vi "Polarity switch.vi"() -> ()   [LabVIEW 2017]
uses:
  <vilib>/DAQmx/write.llb/DAQmx Write (Digital 1D Bool NChan 1Samp 1Line).vi
  <vilib>/DAQmx/miscellaneous.llb/DAQmx Fill In Error Info.vi
  <instrlib>/Keithley KE22xx Series/Keithley KE22xx Series.lvlib
  <instrlib>/Harvard Apparatus PHD Ultra Series/Harvard Apparatus PHD Ultra Series.lvlib
panel:
  in  "Stop acquisition":bool
  in  "Manual selection":enum16{"No control", "Positive", "Negative"}(ring)
  in  "Read volume&time":bool
  out "Volume Units":u16(ring) items=["milliliters", "microliters", "nanoliters", "picoliters"]
  out "Volume":dbl
  in  "Target wait time (min)":dbl
  in  "Count down":bool
  in  "Set harvard pump":bool
  out "error out":errorcluster
  in  "Stop":bool
  in  "Start":bool
  in  "Status":bool
  out "Infusing":bool
  out "Withdrawing":bool
  out "Idle":bool
  in  "Set flow":bool
  in  "Flow Rate (ul/min)":dbl=5.0 format="%#.4f"
  in  "VISA resource name":refnum<visa-resource-name>="COM12"
  in  "New sample":bool
  in  "Sample name":string
  in  "base path":path
  in  "Stop&Save":bool
  in  "Saving data":bool
  out "Sample waiting time (min)":dbl
  out "Current time":timestamp
  out "Start time":timestamp
  in  "Timing":bool
  in  "Read voltage":bool
  out "Waveform Chart":dbl(graph)
  out "Voltage (V)":dbl
  out "Current (mA)":dbl
  in  "Manual Range(0.00)":dbl=3.0 format="%.2f"
  in  "Enable Output":bool
  in  "DC power supply":refnum<visa-resource-name>="USB0::0x05E6::0x2230::9101650::INSTR"
  out "Present (s)":dbl
  in  "stop":bool
  in  "Switching time (s)":dbl
  in  "Start switching":bool
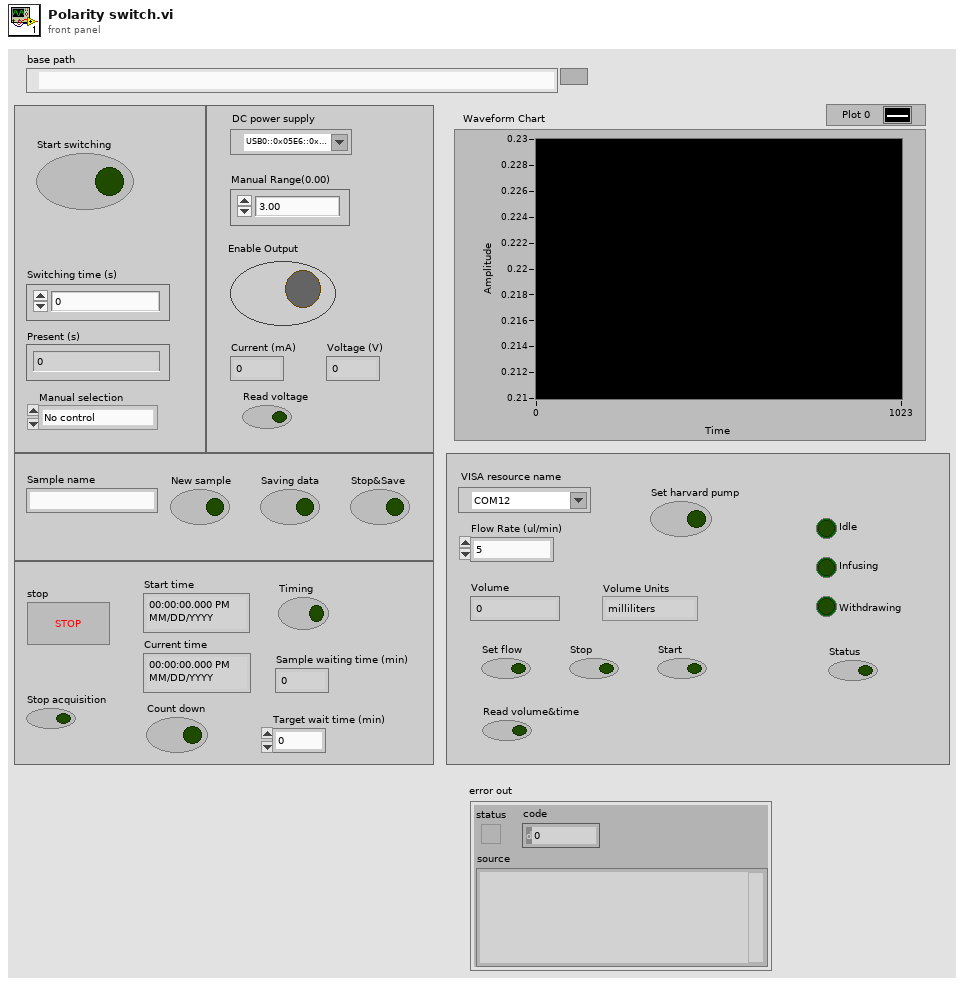
[diagram p1: front panel]
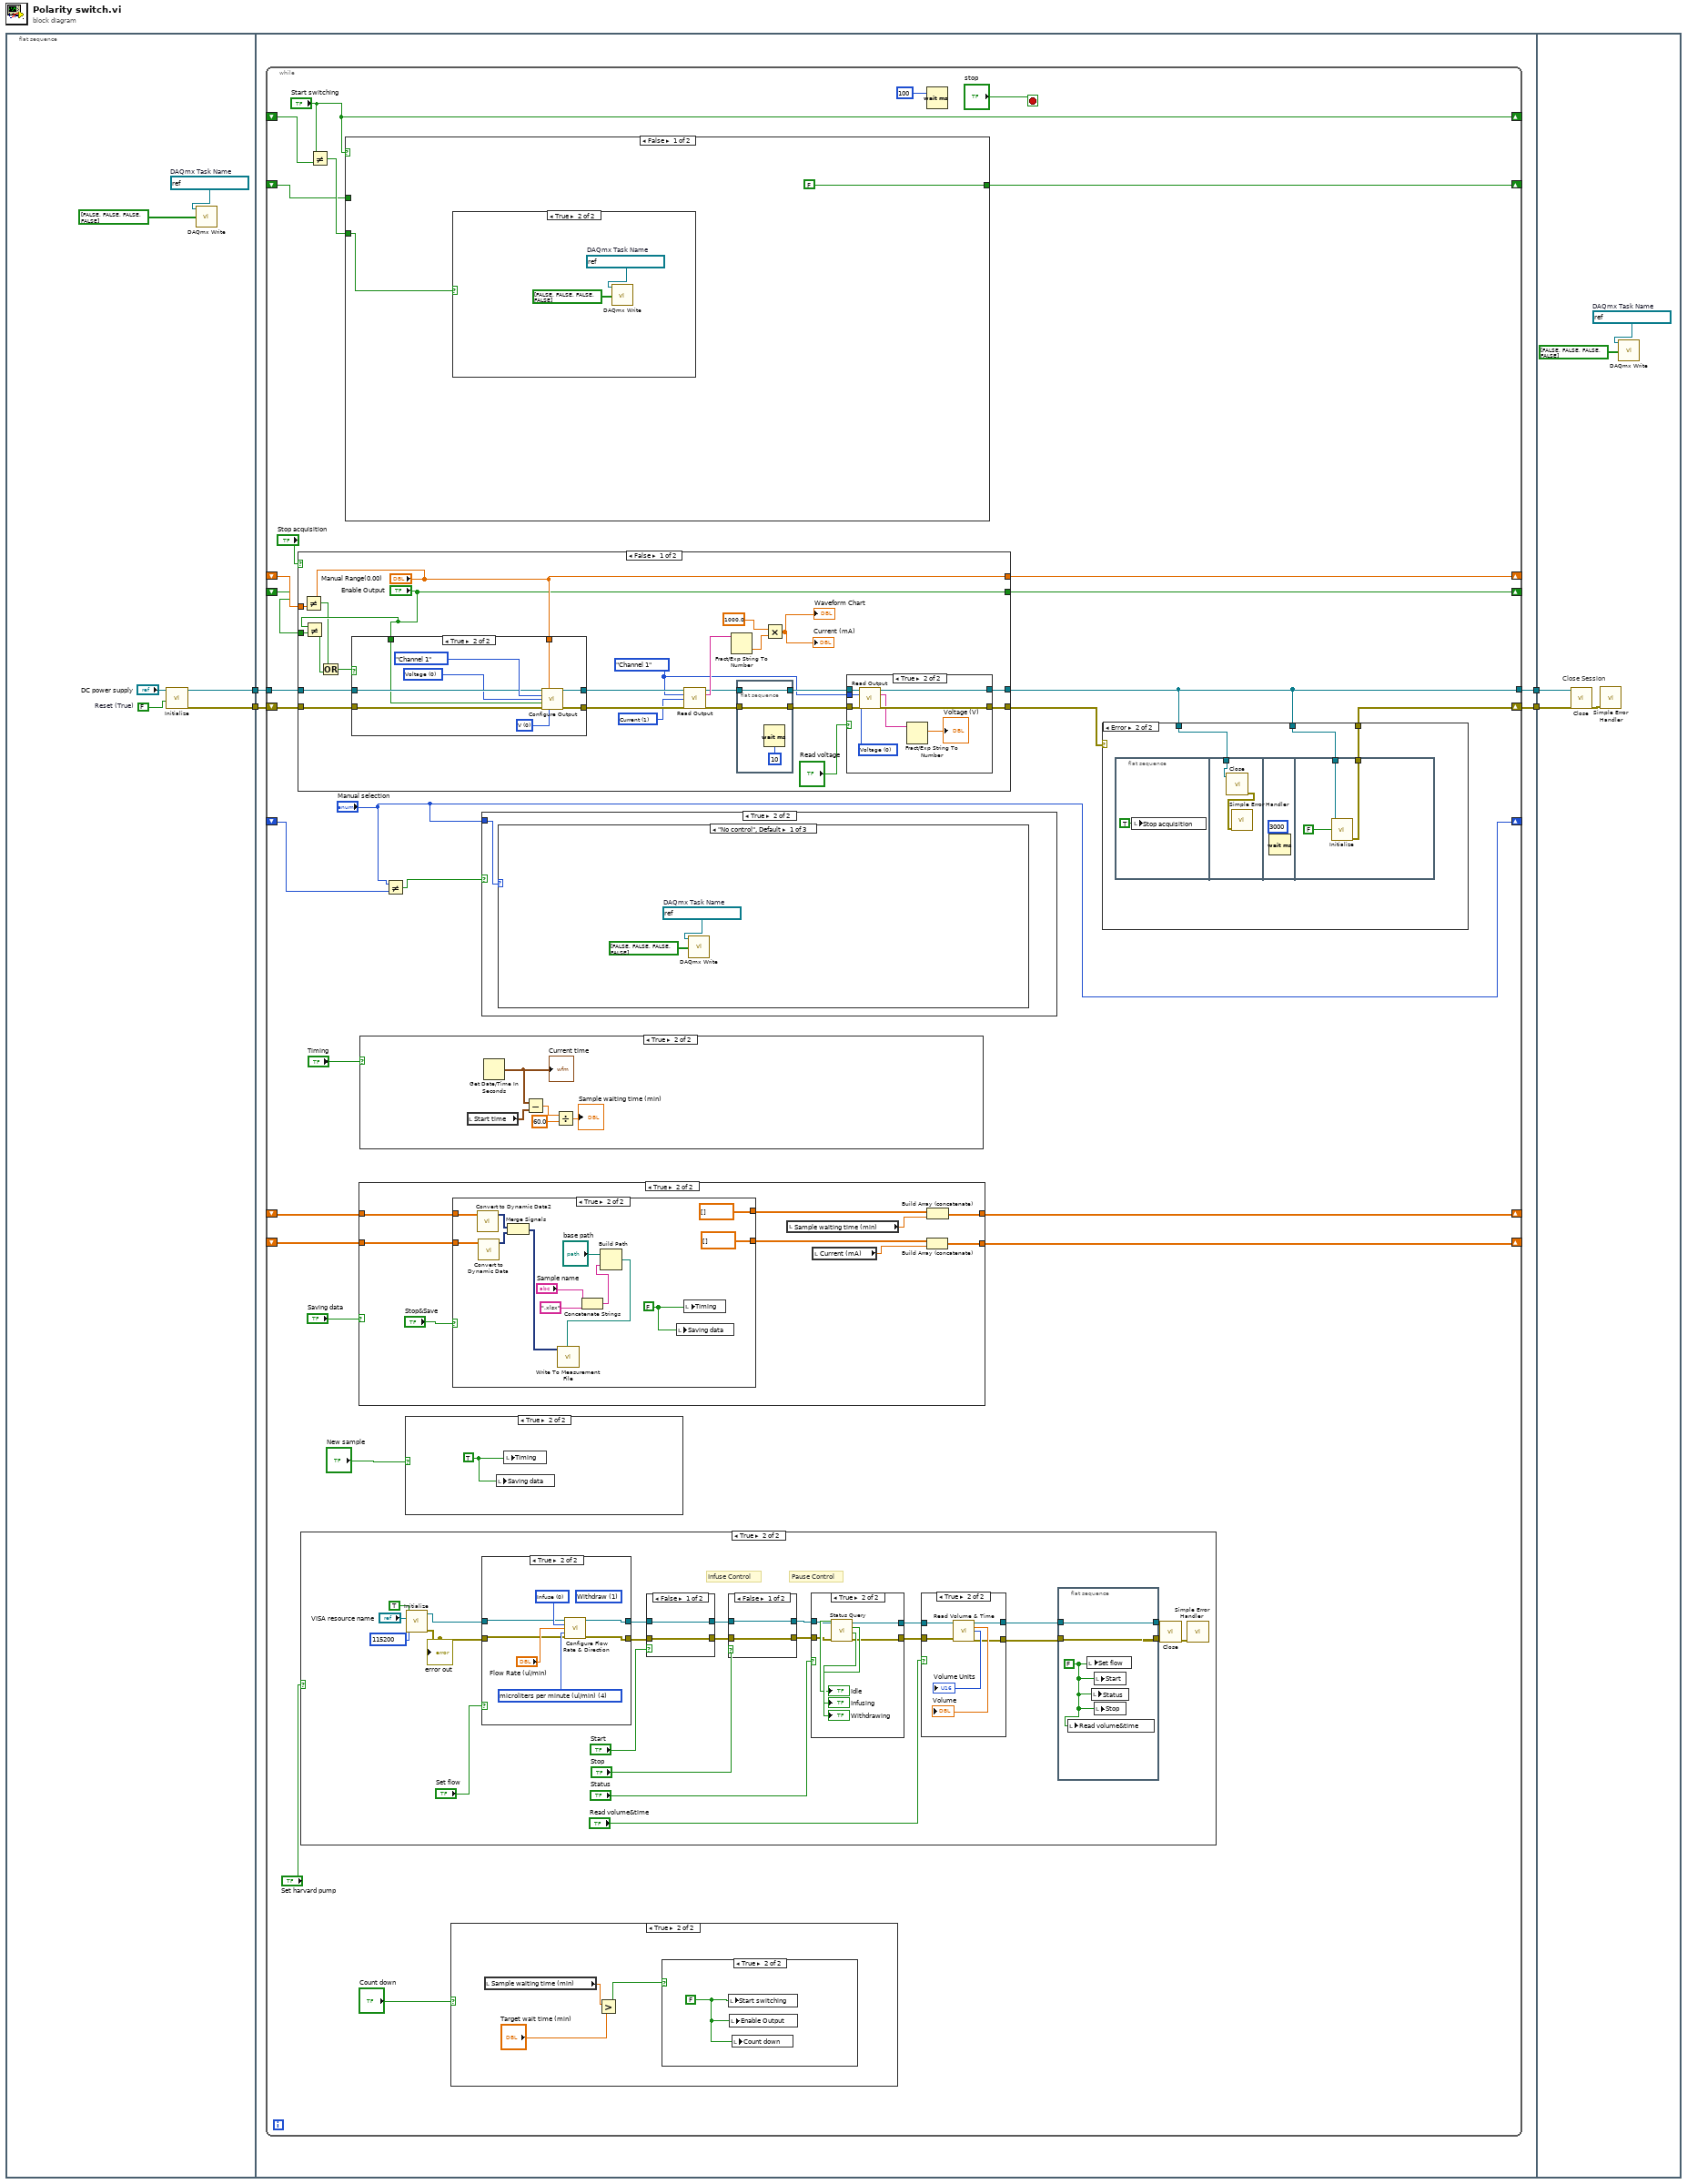
[diagram p0: block diagram]
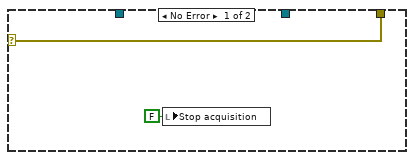
[diagram p5: hidden frame]
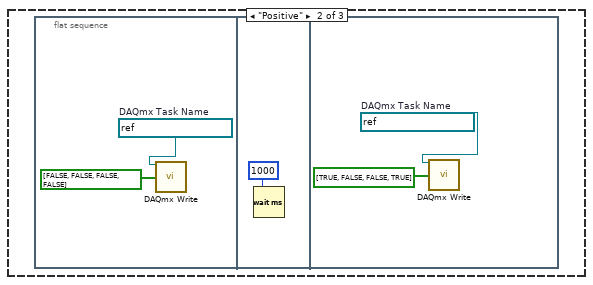
[diagram p7: hidden frame]
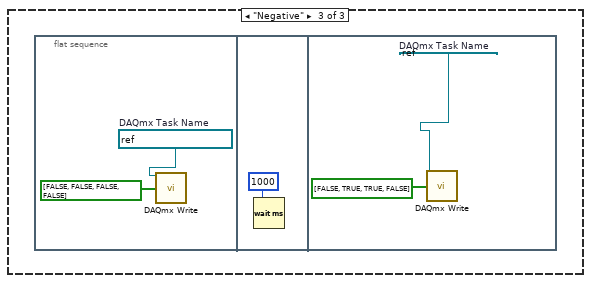
[diagram p8: hidden frame]
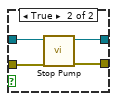
[diagram p15: hidden frame]
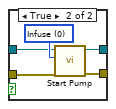
[diagram p16: hidden frame]
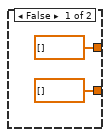
[diagram p18: hidden frame]
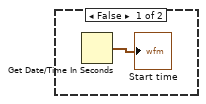
[diagram p20: hidden frame]
diagram:
  n1 = flat-sequence {
    tunnel: [w6] -> w4
    tunnel: [w5] -> w3
    tunnel: w4 -> [w14]
    tunnel: w3 -> [w11]
    tunnel: [w13] -> w2
    tunnel: [w12] -> w1
    tunnel: w2 -> [w248]
    tunnel: w1 -> [w247]
    frame #0 {
      w8 = FALSE items=["OFF", "ON", "OFF", "ON"]  # Reset (True)
      w10 = refnum<k21> "Polarity switch 1"  # DAQmx Task Name
      n2 = call <instrlib>:"Initialize.vi"("Reset (True)"=w8, "VISA resource name"="DC power supply") -> ("error out"=w5:errorcluster, "VISA resource name out"=w6:refnum<visa-resource-name>)  [unwired: 8 in]
      n3 = call-poly <vilib>:"DAQmx Write.vi"("task/channels in"=w10, "data"=bool[] [FALSE, FALSE, FALSE, FALSE]) -> ()  [unwired: 11 in, 3 out]
    }
    frame #1 {
      n4 = while {
        shift-right: ["Start switching"] -> _
        shift-left: _ -> [w42]
        shift-right: [w40] -> _
        shift-left: _ -> [w39]
        tunnel: w14 -> [w36]
        shift-right: [w32] -> _
        shift-left: _ -> [w33]
        shift-right: [w34] -> _
        shift-left: _ -> [w35]
        tunnel: [w18] -> w13
        shift-right: [w29] -> _
        shift-left: _ -> [w27]
        shift-right: [w28] -> _
        shift-left: _ -> [w26]
        shift-right: ["Manual selection"] -> _
        shift-left: _ -> [w21]
        shift-right: [w16] -> w12
        shift-left: w11 -> [w15]
        stop <- "stop" stop-if-true
        n5 = case shown="False" "Stop acquisition" {
          tunnel: w36 -> [w67 w93]
          tunnel: w15 -> [w66 w92]
          tunnel: w35 -> [w65 w95]
          tunnel: ["Manual Range(0.00)" w95] -> w34
          tunnel: w33 -> [w63 w94]
          tunnel: ["Enable Output" w94] -> w32
          tunnel: [w45 w92] -> w19
          tunnel: [w44 w93] -> w18
          frame False {
            w56 = u16 1 items=["Voltage", "Current", "Power"] ("Measurement Function (0:Voltage)")
            w48 = enum16{"Channel 1", "Channel 2", "Channel 3"}."Channel 1" ("Channel Select")
            n6 = Not Equal?(x="Manual Range(0.00)", y=w65) -> (x != y?=w61:bool)
            n7 = Not Equal?(x="Enable Output", y=w63) -> (x != y?=w60:bool)
            n8 = Or(x=w61, y=w60) -> (x .or. y?=w59:bool)
            n9 = case shown="True" w59 {
              tunnel: w67 -> [w82 w90]
              tunnel: w66 -> [w81 w89]
              tunnel: [w81 w87] -> w57
              tunnel: [w82 w86] -> w58
              tunnel: "Manual Range(0.00)" -> [_ w85]
              tunnel: "Enable Output" -> [_ w84]
              frame False {
              }
              frame True {
                w83 = u16 0 items=["Voltage", "Current"] ("Function(0:Voltage)")
                w88 = u16 0 items=["V", "mV", "kV", "A", "mA"] ("Unit(V)")
                n10 = call <instrlib>:"Configure Output.vi"("VISA resource name"=w90, "Manual Range(0.00)"=w85, "Channel Select"=enum16{"Channel 1", "Channel 2", "Channel 3"}."Channel 1", "Function(0:Voltage)"=w83, "Enable Output (T: Enable)"=w84, "error in (no error)"=w89, "Unit(V)"=w88) -> ("VISA resource name out"=w86:refnum<visa-resource-name>, "error out"=w87:errorcluster)  [unwired: 7 in]
              }
            }
            n11 = call <instrlib>:"Read Output.vi"("VISA resource name"=w58, "Channel Select"=w48, "Measurement Function (0:Voltage)"=w56, "error in (no error)"=w57) -> ("VISA resource name out"=w51:refnum<visa-resource-name>, "Measurement"=w55:string, "error out"=w49:errorcluster)  [unwired: 9 in]
            n12 = Fract/Exp String To Number(string=w55) -> (number=w54:dbl)  [unwired: 3 in, 1 out]
            n13 = flat-sequence {
              tunnel: [w80] -> w52
              tunnel: w51 -> [w80]
              tunnel: [w79] -> w50
              tunnel: w49 -> [w79]
              frame #0 {
                n14 = Wait (ms)(milliseconds to wait=u32 10) -> ()  [unwired: 1 out]
              }
            }
            n15 = Multiply(x=1000.0, y=w54) -> (x*y=→"Current (mA)" →"Waveform Chart":dbl)
            n16 = case shown="True" "Read voltage" {
              tunnel: [w69 w76] -> w44
              tunnel: [w68 w75] -> w45
              tunnel: w52 -> [w69 w74]
              tunnel: w50 -> [w68 w73]
              tunnel: w48 -> [_ w72]
              frame False {
              }
              frame True {
                w77 = u16 0 items=["Voltage", "Current", "Power"] ("Measurement Function (0:Voltage)")
                n17 = call <instrlib>:"Read Output.vi"("VISA resource name"=w74, "Channel Select"=w72, "Measurement Function (0:Voltage)"=w77, "error in (no error)"=w73) -> ("VISA resource name out"=w76:refnum<visa-resource-name>, "Measurement"=w70:string, "error out"=w75:errorcluster)  [unwired: 9 in]
                n18 = Fract/Exp String To Number(string=w70) -> (number=→"Voltage (V)":dbl)  [unwired: 3 in, 1 out]
              }
            }
          }
          frame True {
          }
        }
        n19 = case shown="True" "Set harvard pump" {
          frame False {
          }
          frame True {
            w145 = u32 115200 items=["9600"=9600, "19200"=19200, "38400"=38400, "57600"=57600, "115200"=115200] ("Baud Rate (115200)")
            # "Pause Control"
            # "Infuse Control"
            n20 = call <instrlib>:"Initialize.vi"("ID Query (True)"=TRUE, "Baud Rate (115200)"=w145, "VISA resource name"="VISA resource name") -> ("error out"=w140:errorcluster, "VISA resource name out"=w141:refnum<visa-resource-name>)  [unwired: 7 in]
            "error out" <- w140
            n21 = case shown="True" "Set flow" {
              tunnel: w141 -> [w169 w173]
              tunnel: w140 -> [w168 w172]
              tunnel: [w169 w171] -> w139
              tunnel: [w168 w170] -> w138
              frame False {
              }
              frame True {
                w174 = u32 4 items=["milliliters per hour (ml/hr)", "milliliters per minute (ml/min)", "milliliters per second (ml/sec)", "microliters per hour (ul/hr)", "microliters per minute (ul/min)", "microliters per second (ul/sec)", "nanoliters per hour (nl/hr)", "nanoliters per minute (nl/min)", "nanoliters per second (nl/sec)", "picoliters per hour (pl/hr)", "picoliters per minute (pl/min)", "picoliters per second (pl/sec)"] ("Flow Rate Units")
                w176 = u16 0 items=["Infuse", "Withdraw"] ("Pump Method (0:Infuse)")
                (unwired) u16 1 items=["Infuse", "Withdraw"] ("Pump Method (0:Infuse)")
                n22 = call <instrlib>:"Configure Flow Rate & Direction.vi"("VISA resource name"=w173, "Pump Direction (0:Infuse)"=w176, "Flow Rate (5.00)"="Flow Rate (ul/min)", "Flow Rate Units (1:ml/min)"=w174, "error in (no error)"=w172) -> ("VISA resource name out"=w171:refnum<visa-resource-name>, "error out"=w170:errorcluster)  [unwired: 9 in]
              }
            }
            n23 = case shown="False" "Start" {
              tunnel: [w184 w189] -> w144
              tunnel: [w183 w188] -> w143
              tunnel: w139 -> [w184 w186]
              tunnel: w138 -> [w183 w185]
              frame False {
              }
              frame True {
                w187 = u16 0 items=["Infuse", "Withdraw"] ("Run Method (0:Infuse)")
                n24 = call <instrlib>:"Start Pump.vi"("error in (no error)"=w185, "Run Direction (0:Infuse)"=w187, "VISA resource name"=w186) -> ("error out"=w188:errorcluster, "VISA resource name out"=w189:refnum<visa-resource-name>)  [unwired: 7 in]
              }
            }
            n25 = case shown="False" "Stop" {
              tunnel: w144 -> [w178 w182]
              tunnel: w143 -> [w177 w181]
              tunnel: [w178 w180] -> w137
              tunnel: [w177 w179] -> w136
              frame False {
              }
              frame True {
                n26 = call <instrlib>:"Stop Pump.vi"("error in (no error)"=w181, "VISA resource name"=w182) -> ("error out"=w179:errorcluster, "VISA resource name out"=w180:refnum<visa-resource-name>)  [unwired: 8 in]
              }
            }
            n27 = case shown="True" "Status" {
              tunnel: w137 -> [w160 w164]
              tunnel: w136 -> [w159 w163]
              tunnel: [w160 w162] -> w129
              tunnel: [w159 w161] -> w128
              frame False {
              }
              frame True {
                n28 = call <instrlib>:"Status Query.vi"("error in (no error)"=w163, "VISA resource name"=w164) -> ("error out"=w161:errorcluster, "Withdrawing"=→"Withdrawing":bool, "Infusing"=→"Infusing":bool, "VISA resource name out"=w162:refnum<visa-resource-name>, "Idle"=→"Idle":bool)  [unwired: 4 in, 1 out]
              }
            }
            n29 = case shown="True" "Read volume&time" {
              tunnel: w129 -> [w149 w155]
              tunnel: w128 -> [w148 w154]
              tunnel: [w149 w151] -> w127
              tunnel: [w148 w150] -> w126
              frame False {
              }
              frame True {
                n30 = call <instrlib>:"Read Volume & Time .vi"("VISA resource name"=w155, "error in (no error)"=w154) -> ("VISA resource name out"=w151:refnum<visa-resource-name>, "Volume"=→"Volume":dbl, "Volume Units"=→"Volume Units":u16, "error out"=w150:errorcluster)  [unwired: 8 in, 2 out]
              }
            }
            n31 = flat-sequence {
              tunnel: w127 -> [w157]
              tunnel: [w158] -> w132
              tunnel: w126 -> [w158]
              tunnel: [w157] -> w131
              frame #0 {
                w156 = FALSE
                n32 = local write "Read volume&time"(w156) -> ()
                n33 = local write "Set flow"(w156) -> ()
                n34 = local write "Status"(w156) -> ()
                n35 = local write "Start"(w156) -> ()
                n36 = local write "Stop"(w156) -> ()
              }
            }
            n37 = call <instrlib>:"Close.vi"("error in (no error)"=w132, "VISA resource name"=w131) -> ("error out"=w146:errorcluster)  [unwired: 9 in]
            n38 = call <vilib>:"Simple Error Handler.vi"("error in (no error)"=w146) -> ()  [unwired: 4 in, 5 out]
          }
        }
        n39 = Not Equal?(x="Start switching", y=w42) -> (x != y?=w41:bool)
        n40 = case shown="False" "Start switching" {
          tunnel: w41 -> [w223 w227]
          tunnel: [FALSE w231] -> w40
          tunnel: w39 -> [_ w230]
          frame False {
            n41 = case shown="True" w223 {
              frame False {
              }
              frame True {
                w225 = refnum<k21> "Polarity switch 1"  # DAQmx Task Name
                n42 = call-poly <vilib>:"DAQmx Write.vi"("task/channels in"=w225, "data"=bool[] [FALSE, FALSE, FALSE, FALSE]) -> ()  [unwired: 11 in, 3 out]
              }
            }
          }
          frame True {
            n43 = Multiply(x="Switching time (s)", y=2.0) -> (x*y=w233:dbl)
            n44 = call "Elapsed Time"("Time Target (s)"=w233, "Reset"=w227) -> ("Elapsed Time (s)"=w228:dbl)  [unwired: 10 in, 7 out]
            "Present (s)" <- w228
            n45 = Greater?(x="Switching time (s)", y=w228) -> (0:w231:bool)
            n46 = Not Equal?(x=w230, y=w231) -> (x != y?=w229:bool)
            n47 = case shown="False" w231 {
              tunnel: w229 -> [w235 w241]
              frame False {
                n48 = case shown="True" w235 {
                  frame False {
                  }
                  frame True {
                    n49 = flat-sequence {
                      frame #0 {
                        w237 = refnum<k21> "Polarity switch 1"  # DAQmx Task Name
                        n50 = call-poly <vilib>:"DAQmx Write.vi"("task/channels in"=w237, "data"=bool[] [FALSE, FALSE, FALSE, FALSE]) -> ()  [unwired: 11 in, 3 out]
                      }
                      frame #1 {
                        n51 = Wait (ms)(milliseconds to wait=u32 1000) -> ()  [unwired: 1 out]
                      }
                      frame #2 {
                        w239 = refnum<k21> "Polarity switch 1"  # DAQmx Task Name
                        n52 = call-poly <vilib>:"DAQmx Write.vi"("task/channels in"=w239, "data"=bool[] [FALSE, TRUE, TRUE, FALSE]) -> ()  [unwired: 11 in, 3 out]
                      }
                    }
                  }
                }
              }
              frame True {
                n53 = case shown="True" w241 {
                  frame False {
                  }
                  frame True {
                    n54 = flat-sequence {
                      frame #0 {
                        w243 = refnum<k21> "Polarity switch 1"  # DAQmx Task Name
                        n55 = call-poly <vilib>:"DAQmx Write.vi"("task/channels in"=w243, "data"=bool[] [FALSE, FALSE, FALSE, FALSE]) -> ()  [unwired: 11 in, 3 out]
                      }
                      frame #1 {
                        n56 = Wait (ms)(milliseconds to wait=u32 1000) -> ()  [unwired: 1 out]
                      }
                      frame #2 {
                        w245 = refnum<k21> "Polarity switch 1"  # DAQmx Task Name
                        n57 = call-poly <vilib>:"DAQmx Write.vi"("task/channels in"=w245, "data"=bool[] [TRUE, FALSE, FALSE, TRUE]) -> ()  [unwired: 11 in, 3 out]
                      }
                    }
                  }
                }
              }
            }
          }
        }
        n58 = case shown="True" "Saving data" {
          tunnel: [dbl[] [] w201] -> w29
          tunnel: [dbl[] [] w199] -> w28
          tunnel: w27 -> [_ w195]
          tunnel: w26 -> [_ w193]
          frame False {
          }
          frame True {
            n59 = case shown="True" "Stop&Save" {
              tunnel: [w203 dbl[] []] -> w196
              tunnel: w195 -> [w203 w215]
              tunnel: [w202 dbl[] []] -> w194
              tunnel: w193 -> [w202 w216]
              frame False {
              }
              frame True {
                w204 = FALSE ("Timing")
                n60 = call "Convert to Dynamic Data2"("Array"=w215) -> ("Dynamic Data Type"=w214:dynamicdata)  [unwired: 3 in]
                n61 = call "Convert to Dynamic Data"("Array"=w216) -> ("Dynamic Data Type"=w213:dynamicdata)  [unwired: 3 in]
                n62 = Merge Signals(w214, w213) -> (w212:dynamicdata)
                n63 = Concatenate Strings("Sample name", ".xlsx" ("string")) -> (w206:string)
                n64 = Build Path(base path="base path", name or relative path=w206) -> (appended path=w210:path)
                n65 = call "Write To Measurement File"("Signals"=w212, "Filename"=w210) -> ()  [unwired: 15 in, 3 out]
                n66 = local write "Saving data"(w204) -> ()
                n67 = local write "Timing"(w204) -> ()
              }
            }
            n68 = local read "Sample waiting time (min)"() -> (w200:dbl)
            n69 = local read "Current (mA)"() -> (w198:dbl)
            n70 = Build Array (concatenate)(w194, w198) -> (w199:dbl[])
            n71 = Build Array (concatenate)(w196, w200) -> (w201:dbl[])
          }
        }
        n72 = case shown="True" "Timing" {
          frame False {
            n73 = Get Date/Time In Seconds() -> (seconds since 1Jan1904=→"Start time":timestamp)
          }
          frame True {
            n74 = local read "Start time"() -> (w221:timestamp)
            n75 = Get Date/Time In Seconds() -> (seconds since 1Jan1904=w222:timestamp)
            "Current time" <- w222
            n76 = Subtract(x=w222, y=w221) -> (x-y=w219:dbl)
            n77 = Divide(x=w219, y=60.0) -> (x/y=→"Sample waiting time (min)":dbl)
          }
        }
        n78 = Not Equal?(x="Manual selection", y=w21) -> (x != y?=w20:bool)
        n79 = case shown="True" "New sample" {
          frame False {
          }
          frame True {
            w190 = TRUE ("Timing")
            n80 = local write "Saving data"(w190) -> ()
            n81 = local write "Timing"(w190) -> ()
          }
        }
        n82 = case shown="True" "Count down" {
          frame False {
          }
          frame True {
            n83 = local read "Sample waiting time (min)"() -> (w123:dbl)
            n84 = Greater?(x=w123, y="Target wait time (min)") -> (0:w121:bool)
            n85 = case shown="True" w121 {
              frame False {
              }
              frame True {
                w124 = FALSE ("Start switching")
                n86 = local write "Start switching"(w124) -> ()
                n87 = local write "Enable Output"(w124) -> ()
                n88 = local write "Count down"(w124) -> ()
              }
            }
          }
        }
        n89 = case shown="True" w20 {
          tunnel: "Manual selection" -> [_ w108]
          frame False {
          }
          frame True {
            n90 = case shown="\"No control\", Default" w108 {
              frame "No control", Default {
                w109 = refnum<k21> "Polarity switch 1"  # DAQmx Task Name
                n91 = call-poly <vilib>:"DAQmx Write.vi"("task/channels in"=w109, "data"=bool[] [FALSE, FALSE, FALSE, FALSE]) -> ()  [unwired: 11 in, 3 out]
              }
              frame "Positive" {
                n92 = flat-sequence {
                  frame #0 {
                    w112 = refnum<k21> "Polarity switch 1"  # DAQmx Task Name
                    n93 = call-poly <vilib>:"DAQmx Write.vi"("task/channels in"=w112, "data"=bool[] [FALSE, FALSE, FALSE, FALSE]) -> ()  [unwired: 11 in, 3 out]
                  }
                  frame #1 {
                    n94 = Wait (ms)(milliseconds to wait=u32 1000) -> ()  [unwired: 1 out]
                  }
                  frame #2 {
                    w114 = refnum<k21> "Polarity switch 1"  # DAQmx Task Name
                    n95 = call-poly <vilib>:"DAQmx Write.vi"("task/channels in"=w114, "data"=bool[] [TRUE, FALSE, FALSE, TRUE]) -> ()  [unwired: 11 in, 3 out]
                  }
                }
              }
              frame "Negative" {
                n96 = flat-sequence {
                  frame #0 {
                    w117 = refnum<k21> "Polarity switch 1"  # DAQmx Task Name
                    n97 = call-poly <vilib>:"DAQmx Write.vi"("task/channels in"=w117, "data"=bool[] [FALSE, FALSE, FALSE, FALSE]) -> ()  [unwired: 11 in, 3 out]
                  }
                  frame #1 {
                    n98 = Wait (ms)(milliseconds to wait=u32 1000) -> ()  [unwired: 1 out]
                  }
                  frame #2 {
                    w119 = refnum<k21> "Polarity switch 1"  # DAQmx Task Name
                    n99 = call-poly <vilib>:"DAQmx Write.vi"("task/channels in"=w119, "data"=bool[] [FALSE, TRUE, TRUE, FALSE]) -> ()  [unwired: 11 in, 3 out]
                  }
                }
              }
            }
          }
        }
        n100 = Wait (ms)(milliseconds to wait=u32 100) -> ()  [unwired: 1 out]
        n101 = case shown="Error" w19 {
          selector: w19 -> [w97 _]
          tunnel: w18 -> [_ w100]
          tunnel: w18 -> [_ w99]
          tunnel: [w97 w98] -> w16
          frame No Error {
            n102 = local write "Stop acquisition"(FALSE ("Stop acquisition")) -> ()
          }
          frame Error {
            n103 = flat-sequence {
              tunnel: w100 -> [w103]
              tunnel: w99 -> [w107]
              tunnel: [w105] -> w98
              frame #0 {
                n104 = local write "Stop acquisition"(TRUE ("Stop acquisition")) -> ()
              }
              frame #1 {
                n105 = call <instrlib>:"Close.vi"("VISA resource name"=w103) -> ("error out"=w102:errorcluster)  [unwired: 10 in]
                n106 = call <vilib>:"Simple Error Handler.vi"("error in (no error)"=w102) -> ()  [unwired: 1 in, 8 out]
              }
              frame #2 {
                n107 = Wait (ms)(milliseconds to wait=u32 3000) -> ()  [unwired: 1 out]
              }
              frame #3 {
                n108 = call <instrlib>:"Initialize.vi"("Reset (True)"=FALSE ("ID Query (True)"), "VISA resource name"=w107) -> ("error out"=w105:errorcluster)  [unwired: 8 in, 1 out]
              }
            }
          }
        }
      }
    }
    frame #2 {
      w251 = refnum<k21> "Polarity switch 1"  # DAQmx Task Name
      # "Close Session"
      n109 = call <instrlib>:"Close.vi"("error in (no error)"=w247, "VISA resource name"=w248) -> ("error out"=w249:errorcluster)  [unwired: 9 in]
      n110 = call <vilib>:"Simple Error Handler.vi"("error in (no error)"=w249) -> ()  [unwired: 1 in, 8 out]
      n111 = call-poly <vilib>:"DAQmx Write.vi"("task/channels in"=w251, "data"=bool[] [FALSE, FALSE, FALSE, FALSE]) -> ()  [unwired: 11 in, 3 out]
    }
  }
